vi "OMV_Python.vi"(8 "error in (no error)":errorcluster, 10 "Script":string, 11 "Python":T1) -> (0 "error out":errorcluster, 3 "Python":T1)   [LabVIEW 2022 SP3]
uses:
  PythonCtrl.ctl
  Processors.ctl
panel:
  out "Tx":string
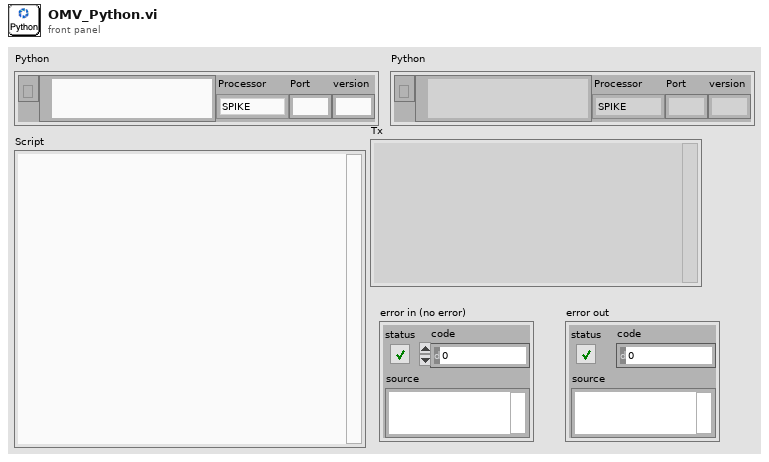
[diagram p1: front panel]
types:
  T1 = typedef "PythonCtrl.ctl" = cluster{"session":refnum<k35>, "PyPath":path, "Processor":T2, "Port":string, "version":string}
  T2 = typedef "Processors.ctl" = enum16{"SPIKE", "Pi", "Pi_ssh", "OpenMV", "Dunio"}
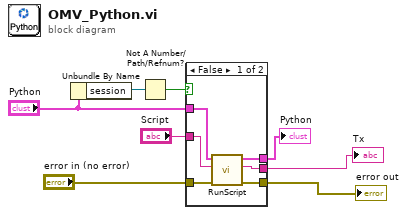
[diagram p0: block diagram]
diagram:
  n1 = Unbundle By Name("Python") -> ("session"=w2:refnum<k35>)
  n2 = Not A Number/Path/Refnum?(number/path/refnum=w2) -> (NaN/Path/Refnum?=w3:bool)
  n3 = case shown="False" w3 {
    tunnel: [w14 w16] -> w8
    tunnel: [w13 w15] -> w7
    tunnel: "Script" -> [w12 _]
    tunnel: "error in (no error)" -> [w11 w15]
    tunnel: "Python" -> [w10 w16]
    tunnel: [w9 _] -> w1
    frame False {
      n4 = call "RunScript.vi"("error in"=w11, "script"=w12, "Python"=w10) -> ("error out"=w13:errorcluster, "Tx"=w9:string, "Python"=w14:T1)  [unwired: 6 in]
    }
    frame True {
    }
  }
  "Python" <- w8
  "error out" <- w7
  "Tx" <- w1
